vi "r_response.vi"(8 "error in (no error)":errorcluster, 11 "response":string) -> (0 "error out":errorcluster, 3 "values":variant[](array[variant]))   [LabVIEW 2017, in "rethinkdb.lvlib"]
uses:
  rethinkdb.lvlib
  914ac796-27b2-451e-b7e8-bb850beead6e.vi
  baeb6880-b455-45bd-8c2a-24346e5095c7.vi
  json_get_names.vi
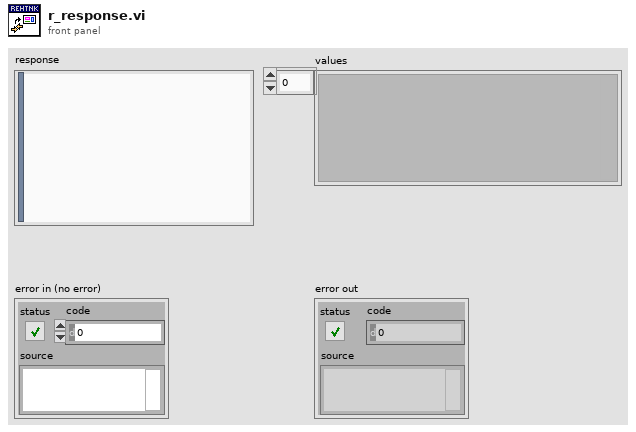
[diagram p1: front panel]
types:
  T1 = typedef "rethinkdb.lvlib/ql2_response.ctl" = enum8{"SUCCESS_ATOM", "SUCCESS_SEQUENCE", "SUCCESS_PARTIAL", "WAIT_COMPLETE", "SERVER_INFO", "CLIENT_ERROR", "COMPILE_ERROR", "RUNTIME_ERROR", "invalid"}
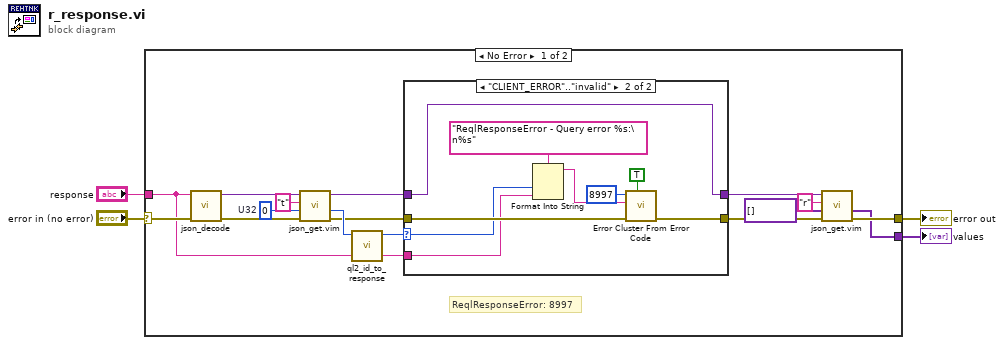
[diagram p0: block diagram]
diagram:
  n1 = case shown="No Error" "error in (no error)" {
    selector: "error in (no error)" -> [w20 w32]
    tunnel: [w9 w32] -> w3
    tunnel: "response" -> [w6 _]
    tunnel: [w5 _] -> w1
    frame No Error {
      w16 = u32 0  # U32
      # "ReqlResponseError: 8997"
      n2 = call "json_decode.vi"("error in (no error)"=w20, "json"=w6) -> ("error out"=w18:errorcluster, "variant"=w19:variant)  [unwired: 8 in]
      n3 = call "json_get.vim"("error in (no error)"=w18, "default"=w16, "name"="t" ("key"), "variant in"=w19) -> ("error out"=w12:errorcluster, "value"=w15:u32, "variant out"=w13:variant)  [unwired: 4 in, 1 out]
      n4 = call "ql2_id_to_response.vi"("id"=w15) -> ("response_type"=w14:T1)  [unwired: 10 in]
      n5 = case shown="\"CLIENT_ERROR\"..\"invalid\"" w14 {
        selector: w14 -> [_ w24]
        tunnel: w13 -> [w21 w31]
        tunnel: w12 -> [w22 w26]
        tunnel: [w22 w25] -> w10
        tunnel: [w21 w31] -> w8
        tunnel: w6 -> [_ w23]
        frame "SUCCESS_ATOM".."SERVER_INFO" {
        }
        frame "CLIENT_ERROR".."invalid" {
          n6 = Format Into String(format string="ReqlResponseError - Query error %s:\n%s" ("error message (\"\")"), w24, w23) -> (resulting string=w30:string)  [unwired: 2 in, 1 out]
          n7 = call <vilib>:"Error Cluster From Error Code.vi"("show call chain? (False)"=TRUE, "error in (no error)"=w26, "error message (\"\")"=w30, "error code (0)"=8997) -> ("error out"=w25:errorcluster)  [unwired: 5 in]
        }
      }
      n8 = call "json_get.vim"("error in (no error)"=w10, "default"=variant[] [], "name"="r" ("key"), "variant in"=w8) -> ("error out"=w9:errorcluster, "value"=w5:variant[])  [unwired: 4 in, 2 out]
    }
    frame Error {
    }
  }
  "error out" <- w3
  "values" <- w1
